vi "Add Waveform Sections.vi"(7 "Names List":bool, 8 "Error In":errorcluster, 9 "External Names":string[](array[string]), 10 "Wfm Pointers":T1[](array[typedef]), 11 "CustomDevice Ref":T2 format="%.0x") -> (0 "Error Out":errorcluster, 3 "CustomDevice Ref":T2 format="%.0x")   [LabVIEW 2017, in "Waveform-Processing-Custom-Device System Explorer.lvlib"]
uses:
  Waveform-Processing-Custom-Device System Explorer.lvlib
  <vilib>/NI Veristand/Custom Device API/Custom Device Item Ref.ctl
  <vilib>/NI Veristand/Custom Device API/Custom Device Pointer.ctl
  NationalInstruments.VeriStand.SystemStorage
  NationalInstruments.VeriStand
  Shared/Constants.vi
  <vilib>/NI Veristand/Custom Device API/Set Item Property (Dependent Node Pointer).vi
  <vilib>/NI VeriStand/Custom Device API/Custom Device API.lvlib
  Shared/Waveform-Processing-Custom-Device Shared.lvlib
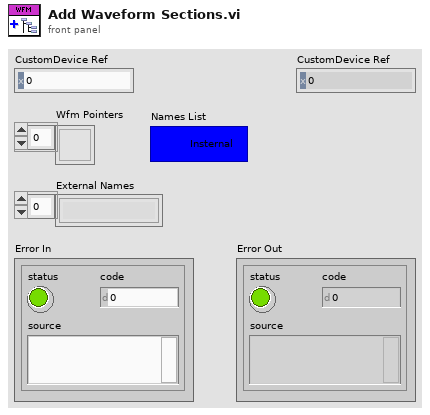
[diagram p1: front panel]
types:
  T1 = typedef "Custom Device API.lvlib/Custom Device Pointer.ctl" = refnum<k24>
  T2 = typedef "Custom Device API.lvlib/Custom Device Item Ref.ctl" = u64
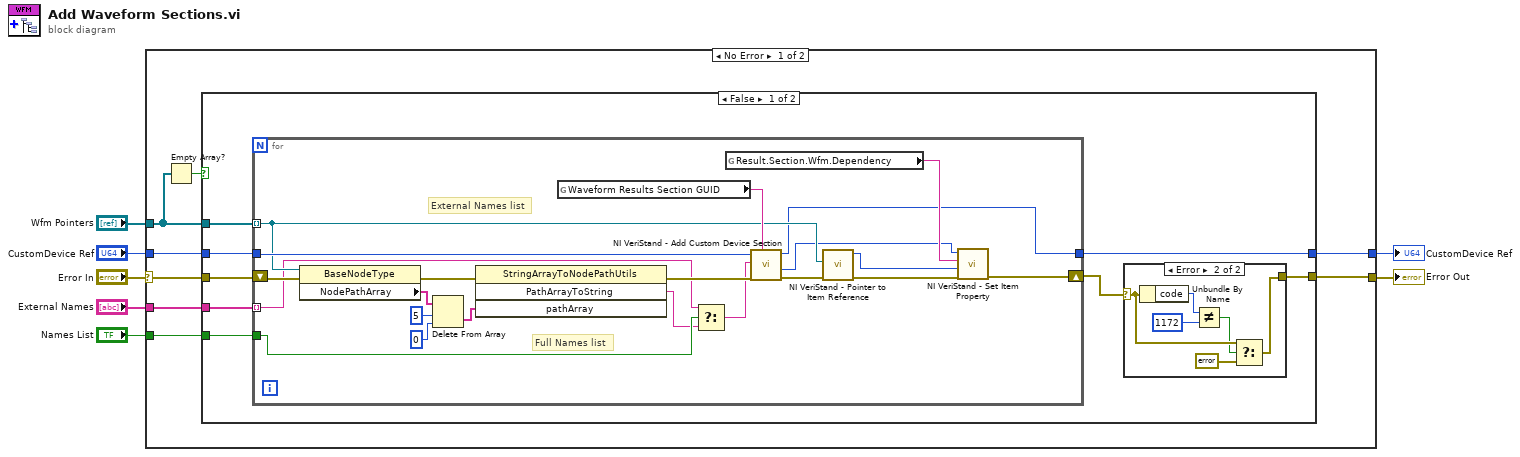
[diagram p0: block diagram]
diagram:
  n1 = case shown="No Error" "Error In" {
    selector: "Error In" -> [w14 w55]
    tunnel: [w13 w55] -> w1
    tunnel: "CustomDevice Ref" -> [w15 w54]
    tunnel: [w12 w54] -> w6
    tunnel: "Wfm Pointers" -> [w11 _]
    tunnel: "External Names" -> [w9 _]
    tunnel: "Names List" -> [w8 _]
    frame No Error {
      n2 = Empty Array?(array=w11) -> (empty?=w10:bool)
      n3 = case shown="False" w10 {
        tunnel: w11 -> [w23 _]
        tunnel: w15 -> [w22 w53]
        tunnel: w14 -> [w21 w52]
        tunnel: [w18 w52] -> w13
        tunnel: [w20 w53] -> w12
        tunnel: w9 -> [w17 _]
        tunnel: w8 -> [w16 _]
        frame False {
          n4 = for {
            tunnel: w22 -> [w44]
            tunnel: w23 -> [w38] mode=indexing
            tunnel: [w34] -> w20
            shift-right: [w35] -> w19
            shift-left: w21 -> [w42]
            tunnel: w17 -> [w28] mode=indexing
            tunnel: w16 -> [w27]
            # "External Names list"
            # "Full Names list"
            n5 = property class="BaseNodeType"(reference=w38, error in=w42) -> (error out=w33:errorcluster, "NodePathArray"=w29:string[])  [unwired: 1 out]
            n6 = Delete From Array(array=w29, length=5, index=0) -> (deleted portion=w26:string[])  [unwired: 1 out]
            n7 = invoke class="StringArrayToNodePathUtils" method="PathArrayToString"(error in=w33, "pathArray"=w26) -> (error out=w32:errorcluster, "PathArrayToString"=w25:string)  [unwired: 2 in, 2 out]
            n8 = global read "Constants.vi" "Waveform Results Section GUID"() -> (w43:string)
            n9 = Select(t=w28, s=w27, f=w25) -> (s? t:f=w24:string)
            n10 = global read "Constants.vi" "Result.Section.Wfm.Dependency"() -> (w41:string)
            n11 = call <vilib>:"NI VeriStand - Add Custom Device Section.vi"("GUID (Default Section)"=w43, "error in (no error)"=w32, "Section Name"=w24, "Parent Ref in"=w44) -> ("error out"=w40:errorcluster, "Section Ptr"=w36:T2, "Parent Ref out"=w34:T2)  [unwired: 4 in, 1 out]
            n12 = call <vilib>:"NI VeriStand - Pointer to Item Reference.vi"("error in (no error)"=w40, "Node Pointer"=w38) -> ("error out"=w39:errorcluster, "Item Ref out"=w37:T2)  [unwired: 8 in]
            n13 = call-poly <vilib>:"NI VeriStand - Set Item Property.vi"("error in (no error)"=w39, "Dependent Node Ref"=w37, "Property Name"=w41, "Item Ref in"=w36) -> ("error out"=w35:errorcluster)  [unwired: 5 in, 2 out]
          }
          n14 = case shown="Error" w19 {
            selector: w19 -> [w45 w49]
            tunnel: [w45 w46] -> w18
            frame No Error {
            }
            frame Error {
              n15 = Unbundle By Name(w49) -> ("code"=w51:i32)
              n16 = Not Equal?(x=w51, y=1172) -> (x != y?=w48:bool)
              n17 = Select(t=w49, s=w48, f=errorcluster {"status"=FALSE, "code"=0, "source"=""}) -> (s? t:f=w46:errorcluster)
            }
          }
        }
        frame True {
        }
      }
    }
    frame Error {
    }
  }
  "CustomDevice Ref" <- w6
  "Error Out" <- w1
